vi "Controlword_CommandToWord.vi"(10 "Device Control Command":T1, 11 "ControlWord In":u16 format="%08b") -> (3 "ControlWord Out":u16 format="%08b")   [LabVIEW 2017, in "WordManipulationLibrary.lvlib"]
uses:
  WordManipulationLibrary.lvlib
  Controlword_Commands.ctl
  Set.vi
  Clear.vi
  Bit Manipulation.lvlib
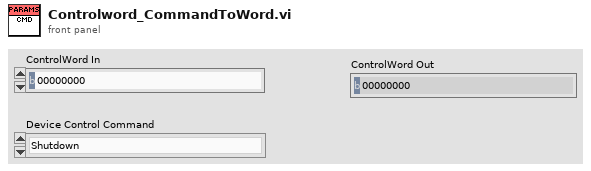
[diagram p1: front panel]
types:
  T1 = typedef "WordManipulationLibrary.lvlib/Controlword_Commands.ctl" = enum16{"Shutdown", "Switch On", "Disable Voltage", "Quick Stop", "Disable Op", "Enable Op", "Fault Reset", "Error"}
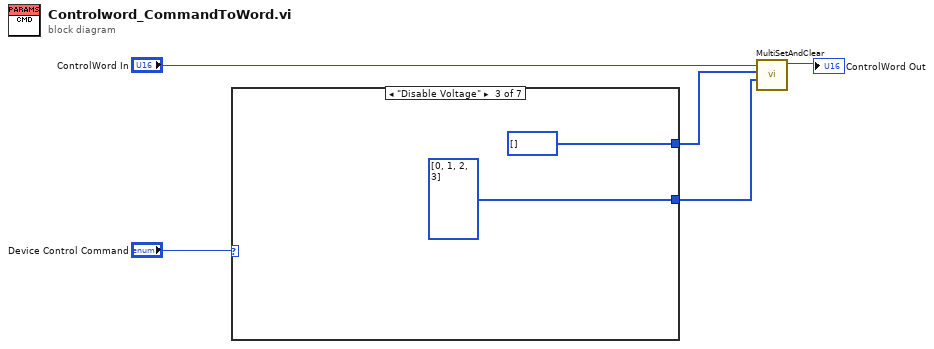
[diagram p0: block diagram]
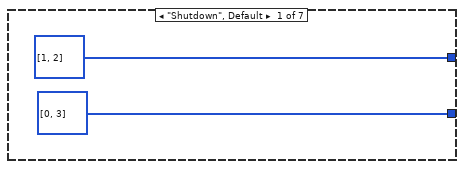
[diagram p2: hidden frame]
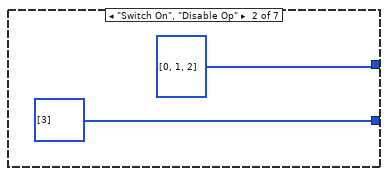
[diagram p3: hidden frame]
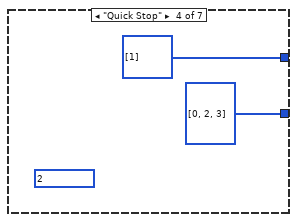
[diagram p4: hidden frame]
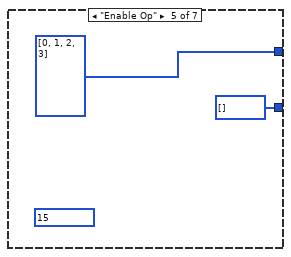
[diagram p5: hidden frame]
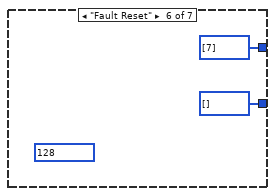
[diagram p6: hidden frame]
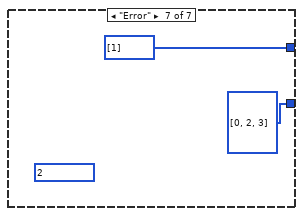
[diagram p7: hidden frame]
diagram:
  n1 = case shown="\"Disable Voltage\"" "Device Control Command" {
    tunnel: [u8[] [1, 2] u8[] [0, 1, 2] ("Bits_To_Clear") u8[] [] ("Bits_To_Clear") u8[] [1] ("Bits_To_Clear") u8[] [0, 1, 2, 3] ("Bits_To_Clear") u8[] [7] ("Bits_To_Clear") u8[] [1] ("Bits_To_Clear")] -> w3
    tunnel: [u8[] [0, 3] u8[] [3] ("Bits_To_Clear") u8[] [0, 1, 2, 3] ("Bits_To_Clear") u8[] [0, 2, 3] ("Bits_To_Clear") u8[] [] ("Bits_To_Clear") u8[] [] ("Bits_To_Clear") u8[] [0, 2, 3] ("Bits_To_Clear")] -> w2
    frame "Shutdown", Default {
    }
    frame "Switch On", "Disable Op" {
    }
    frame "Disable Voltage" {
    }
    frame "Quick Stop" {
      (unwired) u16 2
    }
    frame "Enable Op" {
      (unwired) u16 15
    }
    frame "Fault Reset" {
      (unwired) u16 128
    }
    frame "Error" {
      (unwired) u16 2
    }
  }
  n2 = call "MultiSetAndClear.vi"("Bits_To_Clear"=w2, "Bits_To_Set"=w3, "Data_in"="ControlWord In") -> ("Data_Out"=→"ControlWord Out":u16)  [unwired: 8 in]
